vi "Control Panel - Initialize.vi"(6 "Resource":variant, 8 "error in (no error)":errorcluster, 9 "Receiving Queue":refnum<queue>, 10 "Control Panel Path":path, 11 "Plugin Server in":refnum<class "Generic Plugin.lvclass">) -> (0 "error out":errorcluster, 3 "Plugin Server out":refnum<class "Generic Plugin.lvclass">)   [LabVIEW 2020, in "RxnRover.lvlib" / "Generic Plugin.lvclass"]
doc: "Initialize the Control Panel at the provided controller path. Waits for the initial \"Process Start\" message, where the controller type the control panel reports must match that of the instantiated controller object, or an error is thrown."
uses:
  Generic Plugin.lvclass
  <userlib>/RxnRover/DynamicReentrant/src/Type Defs/Message.ctl
  Generic Plugin.lvclass/Generic Plugin.ctl
  <userlib>/RxnRover/DynamicReentrant/Dynamic Reentrant.lvlib
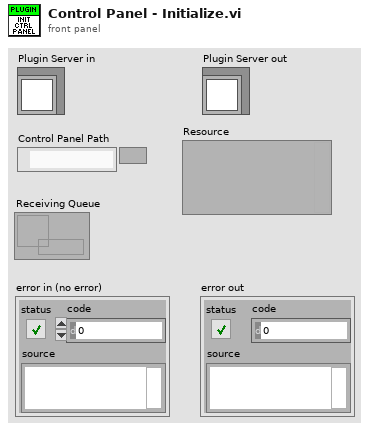
[diagram p1: front panel]
types:
  T1 = typedef "Dynamic Reentrant.lvlib/Message.ctl" = cluster{"Source":string, "Destination":string, "Time Stamp":timestamp, "Command":string, "Data":variant}
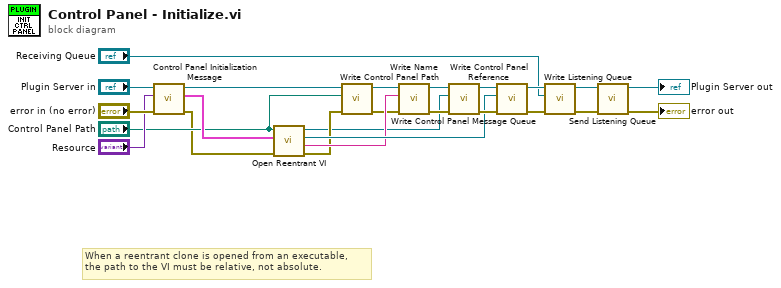
[diagram p0: block diagram]
diagram:
  # "When a reentrant clone is opened from an executable,\nthe path to the VI must be relative, not absolute."
  n1 = call-dynamic "Control Panel Initialization Message.vi"("error in (no error)"="error in (no error)", "Resource"="Resource", "Generic Controller in"="Plugin Server in") -> ("error out"=w1:errorcluster, "Message"=w24:T1, "Generic Controller out"=w4:refnum<class "Generic Plugin.lvclass">)  [unwired: 6 in]
  n2 = call <userlib>:"Open Reentrant VI.vi"("error in (no error)"=w1, "Message"=w24, "VI Path"="Control Panel Path") -> ("error out"=w16:errorcluster, "Clone Name"=w17:string, "VI Refnum"=w20:refnum<vi>, "Reentrant VI Queue"=w9:refnum<queue>)  [unwired: 5 in]
  n3 = call "Write Control Panel Path.vi"("error in (no error)"=w16, "Control Panel Path"="Control Panel Path", "controller in"=w4) -> ("error out"=w5:errorcluster, "controller out"=w3:refnum<class "Generic Plugin.lvclass">)  [unwired: 7 in]
  n4 = call "Write Name.vi"("error in (no error)"=w5, "Name"=w17, "controller in"=w3) -> ("error out"=w21:errorcluster, "controller out"=w18:refnum<class "Generic Plugin.lvclass">)  [unwired: 7 in]
  n5 = call "Write Control Panel Message Queue.vi"("error in (no error)"=w21, "Control Panel.Sending Queue"=w9, "controller in"=w18) -> ("error out"=w22:errorcluster, "controller out"=w19:refnum<class "Generic Plugin.lvclass">)  [unwired: 7 in]
  n6 = call "Write Control Panel Reference.vi"("error in (no error)"=w22, "Reference"=w20, "Generic Controller in"=w19) -> ("error out"=w15:errorcluster, "Generic Controller out"=w12:refnum<class "Generic Plugin.lvclass">)  [unwired: 7 in]
  n7 = call "Write Listening Queue.vi"("error in (no error)"=w15, "Receiving Queue"="Receiving Queue", "Generic Controller in"=w12) -> ("error out"=w11:errorcluster, "Generic Controller out"=w8:refnum<class "Generic Plugin.lvclass">)  [unwired: 7 in]
  n8 = call "Send Listening Queue.vi"("error in (no error)"=w11, "Generic Controller In"=w8) -> ("error out"=→"error out":errorcluster, "Generic Controller Out"=→"Plugin Server out":refnum<class "Generic Plugin.lvclass">)  [unwired: 8 in]
